vi "U3 eDI CR performance tester.vi"() -> (0 "error out":errorcluster)   [LabVIEW 2021]
panel:
  out "Avg ms Per Iteration":dbl format="%.2f"
  out "Total ms":u32
  out "Min Interval":u32
  out "Max Interval":u32
  out "Intervals":u32[](array[numeric])
  in  "Number of Iterations":u32=1000
  in  "stop":bool
  in  "Interval (ms)":u32
  in  "FirstFound":bool=TRUE
  in  "Address":string="1"
  out "Error Message":string
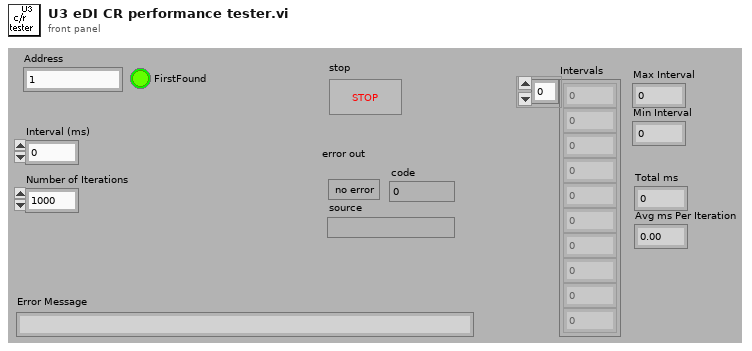
[diagram p1: front panel]
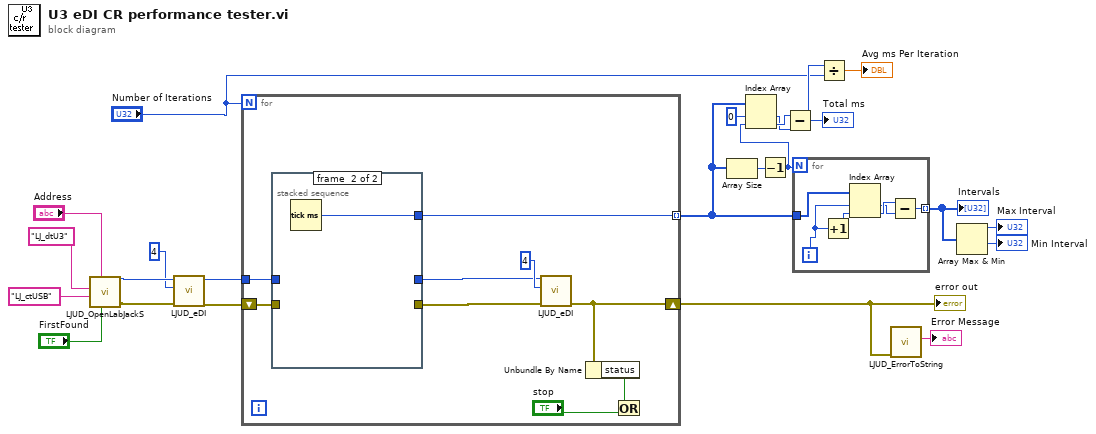
[diagram p0: block diagram]
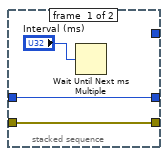
[diagram p2: hidden frame]
diagram:
  n1 = call "LJUD_OpenLabJackS.vi"("FirstFound"="FirstFound", "Address"="Address", "ConnectionType"="LJ_ctUSB", "DeviceType"="LJ_dtU3") -> ("error out"=w14:errorcluster, "Handle"=w15:i32)  [unwired: 5 in, 1 out]
  n2 = call "LJUD_eDI.vi"("error in"=w14, "Channel"=4, "Handle In"=w15) -> ("error out"=w16:errorcluster, "Handle Out"=w17:i32)  [unwired: 6 in, 1 out]
  n3 = for {
    N: "Number of Iterations" -> [_]
    tunnel: w17 -> [w28]
    shift-right: [w30] -> w18
    shift-left: w16 -> [w27]
    tunnel: [w24] -> w8 mode=indexing
    n4 = stacked-sequence {
      tunnel: w28 -> [w33 _]
      tunnel: w27 -> [w34 _]
      tunnel: [w34 _] -> w26
      tunnel: [w33 _] -> w25
      tunnel: [_ w36] -> w24
      frame #0 {
        n5 = Wait Until Next ms Multiple(millisecond multiple="Interval (ms)") -> ()  [unwired: 1 out]
      }
      frame #1 {
        n6 = Tick Count (ms)() -> (millisecond timer value=w36:u32)
      }
    }
    n7 = call "LJUD_eDI.vi"("error in"=w26, "Channel"=4, "Handle In"=w25) -> ("error out"=w30:errorcluster)  [unwired: 6 in, 2 out]
    n8 = Unbundle By Name(w30) -> ("status"=w31:bool)
    n9 = Or(x=w31, y="stop") -> ()  [unwired: 1 out]
  }
  "error out" <- w18
  n10 = Array Size(array=w8) -> (size(s)=w12:i32)
  n11 = Decrement(x=w12) -> (x-1=w6:i32)
  n12 = Index Array(array=w8, index #1=0 ("Index"), index #2=w6) -> (element #1=w1:u32, element #2=w2:u32)
  n13 = Subtract(x=w2, y=w1) -> (x-y=w5:u32)
  "Total ms" <- w5
  n14 = for {
    N: w6 -> [_]
    tunnel: w8 -> [w42]
    tunnel: [w39] -> w11 mode=indexing
    i -> [w40]
    n15 = Increment(x=w40) -> (x+1=w41:i32)
    n16 = Index Array(array=w42, index #1=w40, index #2=w41) -> (element #1=w37:u32, element #2=w38:u32)
    n17 = Subtract(x=w38, y=w37) -> (x-y=w39:u32)
  }
  "Intervals" <- w11
  n18 = Divide(x=w5, y="Number of Iterations") -> (x/y=→"Avg ms Per Iteration":dbl)
  n19 = call "LJUD_ErrorToString.vi"("error in"=w18) -> ("String"=→"Error Message":string)  [unwired: 10 in]
  n20 = Array Max & Min(array=w11) -> (max value=→"Max Interval":u32, min value=→"Min Interval":u32)  [unwired: 2 out]
